vi "Find Main vi path.vi"(11 "Library in":refnum<vi>) -> (2 "Main vi Path":path, 3 "Library out":refnum<vi>)   [LabVIEW 2019, in "Panther Dashboard.lvlib"]
uses:
  Panther Dashboard.lvlib
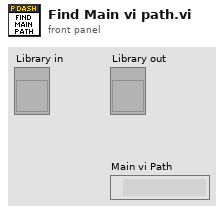
[diagram p1: front panel]
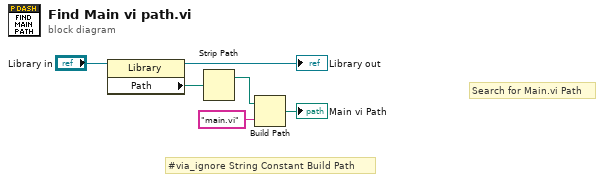
[diagram p0: block diagram]
diagram:
  # "#via_ignore String Constant Build Path"
  # "Search for Main.vi Path"
  n1 = property class="Library"(reference="Library in") -> (reference out=→"Library out":refnum<vi>, "Path"=w3:path)  [unwired: 1 in, 1 out]
  n2 = Strip Path(path=w3) -> (stripped path=w4:path)  [unwired: 1 out]
  n3 = Build Path(base path=w4, name or relative path="main.vi" ("string")) -> (appended path=→"Main vi Path":path)
